vi "读写Excel.vi"   [LabVIEW 2018]
uses:
  <vilib>/Utility/sysdir.llb/System Directory Type.ctl
types:
  T1 = typedef "System Directory Type.ctl" = i32
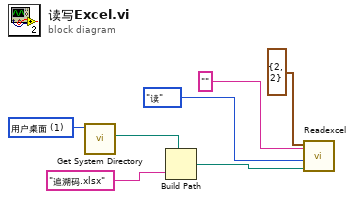
[diagram p0: block diagram]
diagram:
  w7 = T1 1 items=["用户目录"=0, "用户桌面"=1, "用户文档"=2, "用户应用程序数据"=3, "用户设置"=4, "用户临时目录"=5, "公共文档"=6, "公共应用程序数据"=7, "公共设置"=8, "公共缓存"=13, "系统核心库"=9, "系统安装库"=10, "应用程序文件"=11, "启动盘根目录"=12] ("system directory type")
  n1 = call <vilib>:"Get System Directory.vi"("system directory type"=w7) -> ("system directory"=w6:path)  [unwired: 10 in]
  n2 = Build Path(base path=w6, name or relative path="追溯码.xlsx" ("名称或相对路径")) -> (appended path=w4:path)
  n3 = call "Readexcel.vi"(7:"" ("formula"), 8:w4, 9:enum16{"", "写", "读"}."读" ("枚举"), 11:cluster{"row":i32, "column":i32} {"row"=2, "column"=2} ("start (0, 0)")) -> ()  [unwired: 7 in, 1 out]
